vi "choosePath.vi"(8 "error in (no error)":errorcluster, 11 "Pixelfly in":refnum<class "Pixelfly.lvclass">) -> (0 "error out":errorcluster, 2 "Path":path, 3 "Pixelfly out":refnum<class "Pixelfly.lvclass">)   [LabVIEW 2009, in "Hardware.lvlib" / "Channels.lvlib" / "Pixelfly.lvclass"]
uses:
  Pixelfly.lvclass
  Pixelfly.lvclass/Pixelfly.ctl
  Camera.lvclass
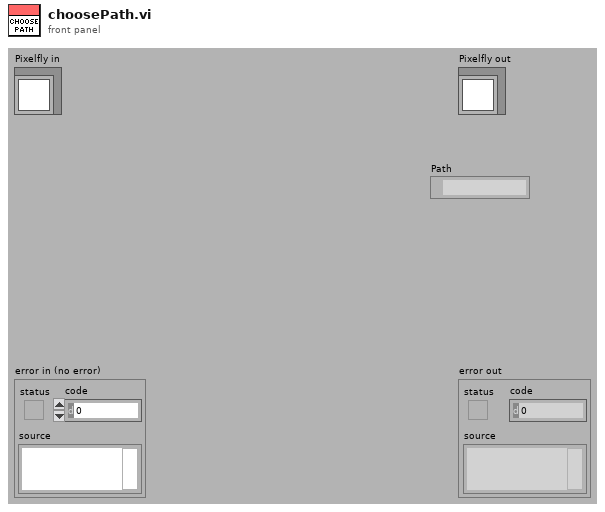
[diagram p1: front panel]
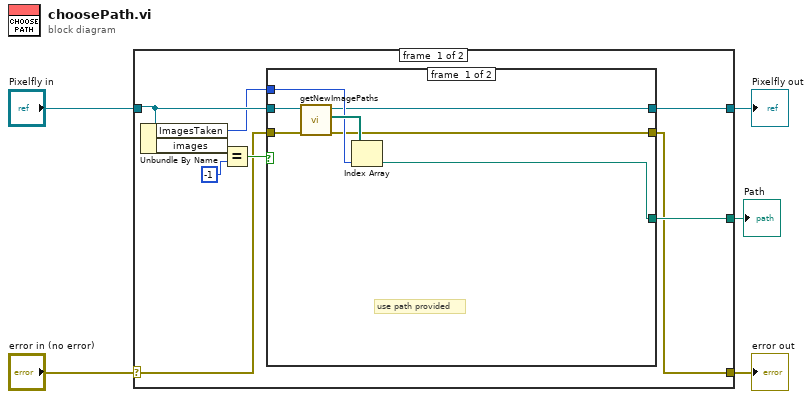
[diagram p0: block diagram]
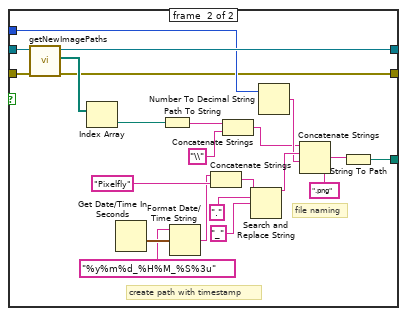
[diagram p2: hidden frame]
diagram:
  n1 = case shown="No Error" "error in (no error)" {
    selector: "error in (no error)" -> [w9 w45]
    tunnel: [w6 w45] -> w4
    tunnel: [w13 w44] -> w2
    tunnel: "Pixelfly in" -> [w14 w44]
    tunnel: [w7 _] -> w1
    frame #0 {
      n2 = Unbundle By Name(w14) -> ("ImagesTaken"=w8:i32, "images"=w12:i32)
      n3 = Equal?(x=w12, y=-1) -> (x = y?=w10:bool)
      n4 = case shown="True" w10 {
        tunnel: w14 -> [w21 w31]
        tunnel: [w17 w30] -> w13
        tunnel: w9 -> [w20 w29]
        tunnel: w8 -> [w18 w28]
        tunnel: [w16 w26] -> w6
        tunnel: [w15 w24] -> w7
        frame #0 {
          # "use path provided"
          n5 = call "getNewImagePaths.vi"("error in (no error)"=w20, "Camera in"=w21) -> ("error out"=w16:errorcluster, "ImagePaths"=w19:path[], "Camera out"=w17:refnum<class "Pixelfly.lvclass">)  [unwired: 7 in]
          n6 = Index Array(array=w19, index=w18) -> (element=w15:path)
        }
        frame #1 {
          # "create path with timestamp"
          # "file naming"
          n7 = call "getNewImagePaths.vi"("error in (no error)"=w29, "Camera in"=w31) -> ("error out"=w26:errorcluster, "ImagePaths"=w27:path[], "Camera out"=w30:refnum<class "Pixelfly.lvclass">)  [unwired: 7 in]
          n8 = Index Array(array=w27) -> (element=w22:path)  [unwired: 1 in]
          n9 = Get Date/Time In Seconds() -> (seconds since 1Jan1904=w42:timestamp)
          n10 = Path To String(path=w22) -> (string=w23:string)
          n11 = Format Date/Time String(time format string (%c)="%y%m%d_%H%M_%S%3u", seconds (now)=w42) -> (date/time string=w40:string)  [unwired: 1 in]
          n12 = Concatenate Strings(w40, "Pixelfly") -> (w39:string)
          n13 = Concatenate Strings(w23, "\\") -> (w32:string)
          n14 = Search and Replace String(input string=w39, search string=".", replace string="_") -> (result string=w35:string)  [unwired: 5 in, 3 out]
          n15 = Number To Decimal String(number=w28) -> (decimal integer string=w34:string)  [unwired: 1 in]
          n16 = Concatenate Strings(w32, w35, w34, ".png") -> (w25:string)
          n17 = String To Path(string=w25) -> (path=w24:path)
        }
      }
    }
    frame #1 {
    }
  }
  "error out" <- w4
  "Pixelfly out" <- w2
  "Path" <- w1
